vi "ShowDepthMap.vi"(2 "error in (no error)":errorcluster, 3 "DepthMap Reference in":refnum<k24>) -> (0 "2D Image out":T1, 1 "error out":errorcluster)   [LabVIEW 2023]
uses:
  C:/Program Files/National Instruments/LabVIEW 2025/MechEyeApiNet.dll
  Program Files/National Instruments/LabVIEW 2025/MechEyeApiNet.dll
  <vilib>/vision/Image Controls.llb/IMAQ Image.ctl
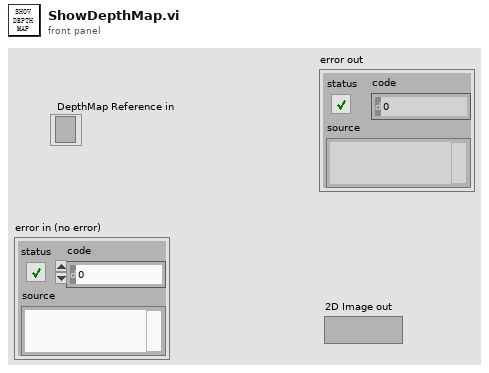
[diagram p1: front panel]
types:
  T1 = typedef "IMAQ Image.ctl" = refnum<image>
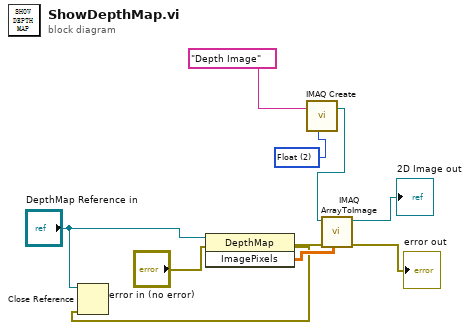
[diagram p0: block diagram]
diagram:
  w9 = u32 2 items=["8 bits", "16 bits", "Float", "Complex", "RGB", "HSL"] ("Image Type")
  n1 = invoke class="DepthMap" method="ImagePixels"(reference="DepthMap Reference in", error in="error in (no error)") -> (error out=w2:errorcluster, "ImagePixels"=w3:sgl[][])  [unwired: 1 in, 1 out]
  n2 = Close Reference(reference="DepthMap Reference in", error in (no error)=w2) -> ()  [unwired: 1 out]
  n3 = call "IMAQ Create"("Image Name"="Depth Image", "Image Type"=w9) -> ("New Image"=w6:T1)  [unwired: 3 in, 1 out]
  n4 = call "IMAQ ArrayToImage"("Image Pixels (Float)"=w3, "error in (no error)"=w2, "Image"=w6) -> ("error out"=→"error out":errorcluster, "Image Out"=→"2D Image out":T1)  [unwired: 7 in]
